vi "Test Write Numpy Array.vi"() -> ()   [LabVIEW 2013]
uses:
  PyLab.lvlib
panel:
  in  "Zip Path":path=path "C:/Users/plane/Desktop/fart.npz"
  in  "Array 1 Path":path=path "C:/Users/plane/Desktop/array_1.npy"
  in  "Array 0 Path":path=path "C:/Users/plane/Desktop/array_0.npy"
  in  "Array":dbl[][](array[numeric])=[[1.0, 2.0, 3.0], [4.0, 5.0, 6.0], [7.0, 8.0, 9.0]]
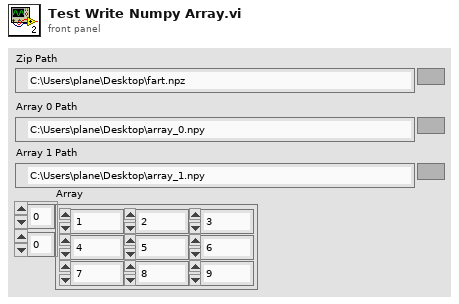
[diagram p1: front panel]
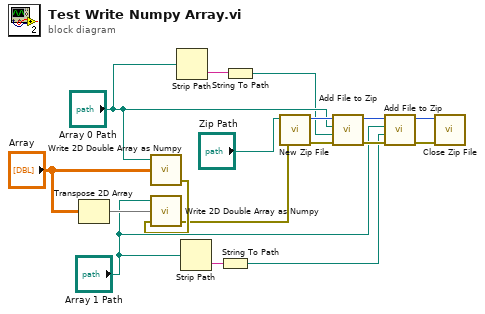
[diagram p0: block diagram]
diagram:
  n1 = Transpose 2D Array(2D array="Array") -> (transposed array=w14:dbl[][])
  n2 = call "Write 2D Double Array as Numpy.vi"("Array"="Array", "Path"="Array 0 Path") -> ("error out"=w6:errorcluster)  [unwired: 3 in]
  n3 = call "Write 2D Double Array as Numpy.vi"("error in"=w6, "Array"=w14, "Path"="Array 1 Path") -> ("error out"=w5:errorcluster)  [unwired: 2 in]
  n4 = Strip Path(path="Array 0 Path") -> (name=w4:string)  [unwired: 1 out]
  n5 = Strip Path(path="Array 1 Path") -> (name=w2:string)  [unwired: 1 out]
  n6 = String To Path(string=w2) -> (path=w1:path)
  n7 = String To Path(string=w4) -> (path=w3:path)
  n8 = call <vilib>:"New Zip File.vi"("error in (no error)"=w5, "target"="Zip Path") -> ("error out"=w17:errorcluster, "zip file out"=w16:i64)  [unwired: 3 in, 1 out]
  n9 = call <vilib>:"Add File to Zip.vi"("error in (no error)"=w17, "destination path in zip"=w3, "source file path"="Array 0 Path", "zip file in"=w16) -> ("error out"=w13:errorcluster, "zip file out"=w12:i64)  [unwired: 6 in]
  n10 = call <vilib>:"Add File to Zip.vi"("error in (no error)"=w13, "destination path in zip"=w1, "source file path"="Array 1 Path", "zip file in"=w12) -> ("error out"=w10:errorcluster, "zip file out"=w11:i64)  [unwired: 6 in]
  n11 = call <vilib>:"Close Zip File.vi"("error in (no error)"=w10, "zip file in"=w11) -> ()  [unwired: 5 in, 1 out]
